vi "Find Abberation Excel Files_SLM.vi"() -> (0 "Ring Menu":cluster{"result string":string, i32}[](array[cluster]), 3 "Abberation File Paths":path[](array[path]))   [LabVIEW 2018]
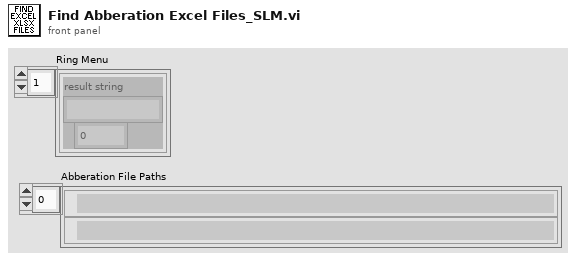
[diagram p1: front panel]
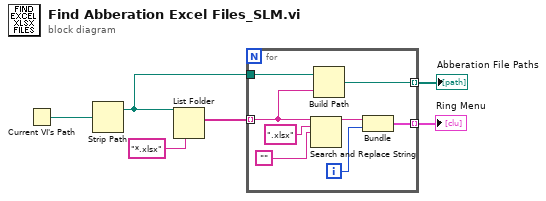
[diagram p0: block diagram]
diagram:
  n1 = Current VI's Path() -> (path=w1:path)
  n2 = Strip Path(path=w1) -> (stripped path=w2:path)  [unwired: 1 out]
  n3 = List Folder(path=w2, pattern="*.xlsx") -> (filenames=w6:string[])  [unwired: 2 in, 3 out]
  n4 = for {
    tunnel: w6 -> [w8] mode=indexing
    tunnel: [w10] -> w5 mode=indexing
    tunnel: w2 -> [w9]
    tunnel: [w7] -> w4 mode=indexing
    i -> [w11]
    n5 = Search and Replace String(input string=w8, search string=".xlsx", replace string="") -> (result string=w12:string)  [unwired: 5 in, 3 out]
    n6 = Build Path(base path=w9, name or relative path=w8) -> (appended path=w7:path)
    n7 = Bundle("result string"=w12, w11) -> (w10:cluster{"result string":string, i32})  [unwired: 1 in]
  }
  "Ring Menu" <- w5
  "Abberation File Paths" <- w4
